vi "Day 4 - Scratchcards.vi"() -> ()   [LabVIEW 2020, in "AoC 2023.lvlib"]
uses:
  AoC 2023.lvlib
  <vilib>/Utility/miscctls.llb/LVMapReplaceAction.ctl
  0a7cd956-c678-4c40-ba95-56d0818c301c.vi
  3b086681-bc74-48f0-999b-988c14eea146.vi
  9d519f65-ef92-499d-aef6-91ab72298a4b.vi
  0a7cd956-c678-4c40-ba95-56d0818c301c.vi/7c7783df-fd5a-49d9-9b7a-63cc9fb0e4e5.vi
  3b086681-bc74-48f0-999b-988c14eea146.vi/7c7783df-fd5a-49d9-9b7a-63cc9fb0e4e5.vi
panel:
  out "Puzzle Part-2 Answer":string
  out "Puzzle Answer":string
  in  "Puzzle Input":string="Card 1: 41 48 83 86 17 | 83 86  6 31 17  9 48 53\nCard 2: 13 32 20 16 61 | 61 30 68 82 17 32 24 19\nCard 3:  1 21 53 59 44 | 69 82 63 72 16 21 14  1\nCard 4: 41 92 73 84 69 | 59 84 76 51 58  5 54 83\nCard 5: 87 83 26 28 32 | 88 30 70 12 93 22 82 36\nCard 6: 31 18 13 56 72 | 74 77 10 23 35 67 36 11"
  # "Enter the Puzzle Input and run the VI"
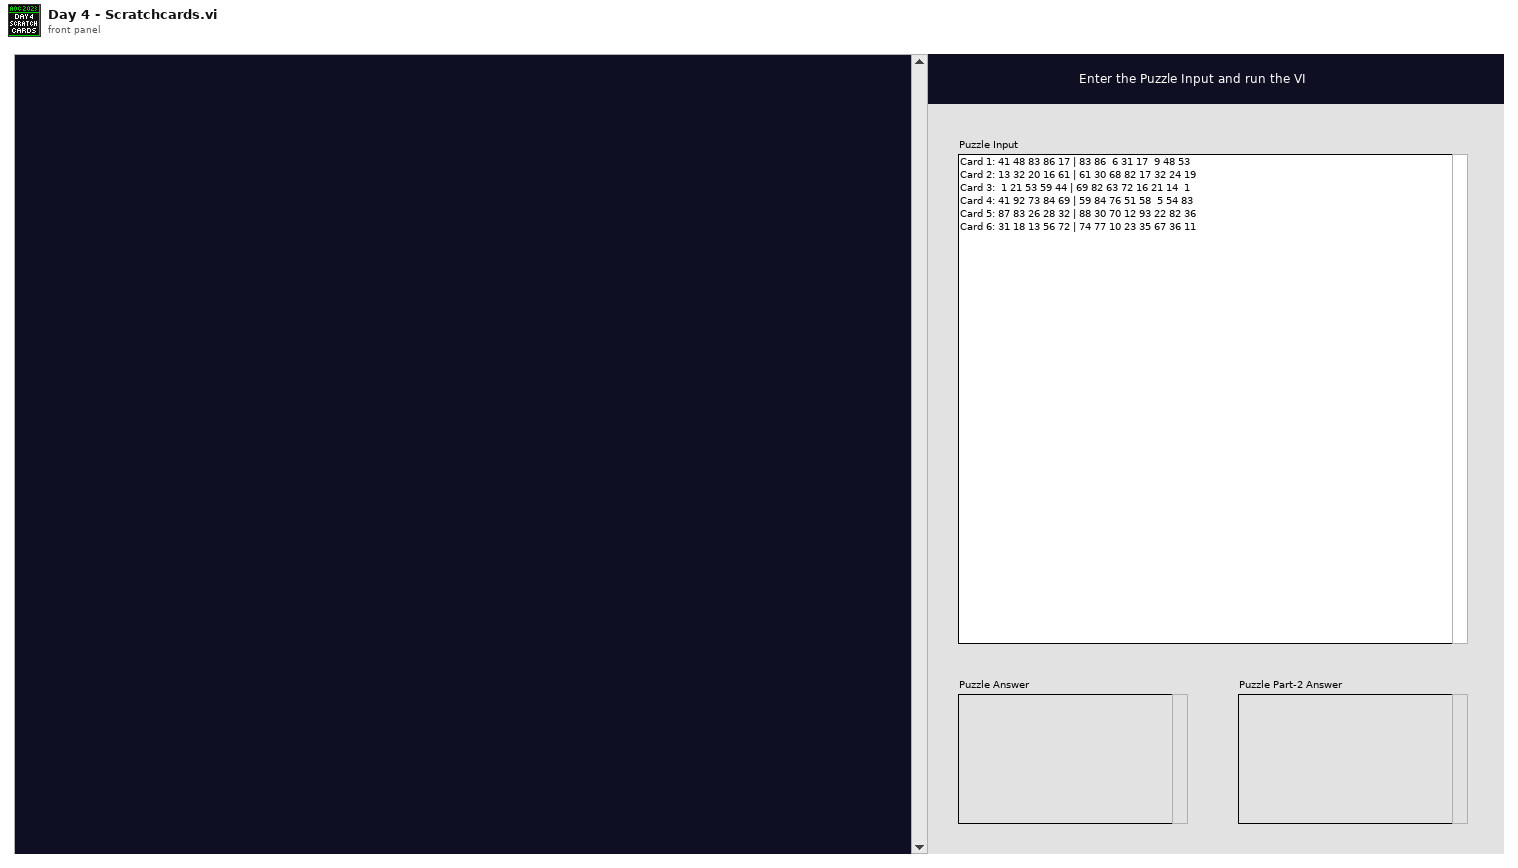
[diagram p1: front panel]
types:
  T1 = typedef "LVMapReplaceAction.ctl" = enum32{"Modify Entry only if found", "Add or Modify Entry", "Delete Entry"}
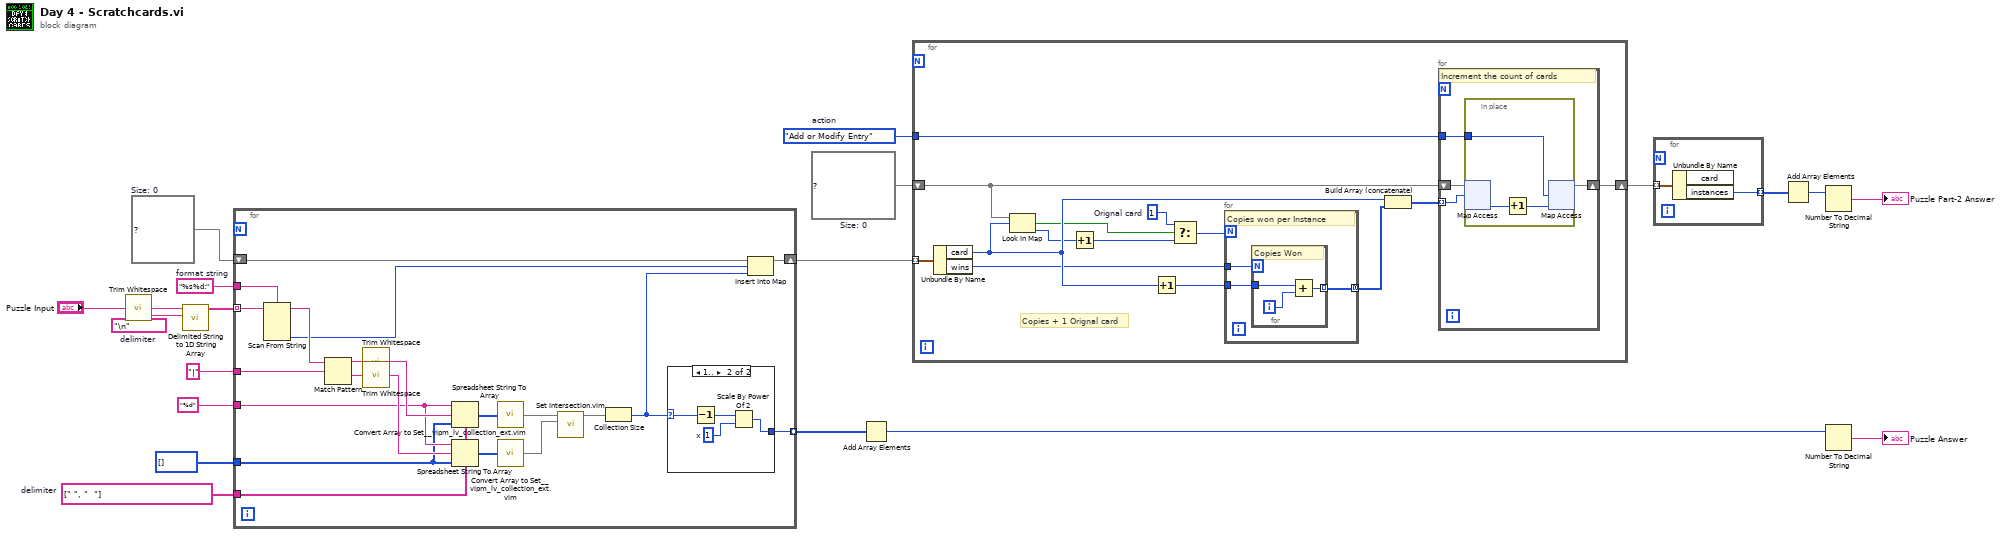
[diagram p0: block diagram]
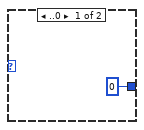
[diagram p2: hidden frame]
diagram:
  w1 = string[] [" ", "  "]  # delimiter
  w5 = map{i32, i32} {}  # Size: 0
  w6 = LVMapReplaceAction."Add or Modify Entry"  # action
  w8 = map{i32, i32} {}  # Size: 0
  w9 = "%s%d:"  # format string
  w17 = "\n"  # delimiter
  n1 = call <vilib>:"Trim Whitespace.vi"("string"="Puzzle Input") -> ("trimmed string"=w16:string)  [unwired: 1 in]
  n2 = call <vilib>:"Delimited String to 1D String Array.vi"("delimiter"=w17, "delimited string"=w16) -> ("string array"=w15:string[])  [unwired: 9 in]
  n3 = for {
    tunnel: w15 -> [w27] mode=indexing
    tunnel: "|" -> [w41]
    tunnel: "%d" -> [w31]
    shift-right: [w38] -> w7
    shift-left: w8 -> [w37]
    tunnel: [w34] -> w12 mode=indexing
    tunnel: i32[] [] -> [w30]
    tunnel: w9 -> [w26]
    tunnel: w1 -> [w21]
    n4 = Scan From String(format string=w26, input string=w27) -> (remaining string=w25:string, output 2=w22:i32)  [unwired: 5 in, 2 out]
    n5 = Match Pattern(string=w25, regular expression=w41) -> (before substring=w40:string, after substring=w39:string)  [unwired: 1 in, 2 out]
    n6 = call <vilib>:"Trim Whitespace.vi"("string"=w40) -> ("trimmed string"=w33:string)  [unwired: 1 in]
    n7 = call <vilib>:"Trim Whitespace.vi"("string"=w39) -> ("trimmed string"=w32:string)  [unwired: 1 in]
    n8 = Spreadsheet String To Array(delimiter (Tab)=w21, format string=w31, spreadsheet string=w33, array type (2D Dbl)=w30) -> (array=w29:i32[])
    n9 = Spreadsheet String To Array(delimiter (Tab)=w21, format string=w31, spreadsheet string=w32, array type (2D Dbl)=w30) -> (array=w28:i32[])
    n10 = call "Convert Array to Set__vipm_lv_collection_ext.vim"("array"=w29) -> ("set"=w36:set{i32})  [unwired: 6 in]
    n11 = call "Convert Array to Set__vipm_lv_collection_ext.vim"("array"=w28) -> ("set"=w35:set{i32})  [unwired: 6 in]
    n12 = call "Set Intersection.vim"("set 2"=w35, "set 1"=w36) -> ("intersection"=w24:set{i32})  [unwired: 9 in]
    n13 = Collection Size(1:w24) -> (0:w23:i32)
    n14 = case shown="1.." w23 {
      selector: w23 -> [_ w44]
      tunnel: [0 w46] -> w34
      frame ..0 {
      }
      frame 1.. {
        w45 = 1  # x
        n15 = Decrement(x=w44) -> (x-1=w43:i32)
        n16 = Scale By Power Of 2(n=w43, x=w45) -> (x*2^n=w46:i32)
      }
    }
    n17 = Insert Into Map(map in=w37, key=w22, value=w23) -> (map out=w38:map{i32, i32})  [unwired: 2 out]
  }
  n18 = Add Array Elements(numeric array=w12) -> (sum=w11:i32)
  n19 = for {
    tunnel: w7 -> [w60] mode=indexing
    tunnel: w6 -> [w59]
    shift-right: [w58] -> w4
    shift-left: w5 -> [w54]
    w49 = 1  # Orignal card
    # "Copies + 1 Orignal card"
    n20 = Unbundle By Name(w60) -> ("card"=w53:i32, "wins"=w52:i32)
    n21 = Look In Map(map=w54, key=w53) -> (key not found?=w50:bool, value=w48:i32)  [unwired: 1 in]
    n22 = Increment(x=w48) -> (x+1=w47:i32)
    n23 = Increment(x=w53) -> (x+1=w57:i32)
    n24 = Select(t=w49, s=w50, f=w47) -> (s? t:f=w51:i32)
    n25 = for {
      N: w51 -> [_]
      tunnel: w57 -> [w63]
      tunnel: [w62] -> w56 mode=concatenating
      tunnel: w52 -> [w61]
      # "Copies won per Instance"
      n26 = for {
        N: w61 -> [_]
        tunnel: w63 -> [w66]
        tunnel: [w64] -> w62 mode=indexing
        i -> [w65]
        # "Copies Won"
        n27 = Add(x=w66, y=w65) -> (x+y=w64:i32)
      }
    }
    n28 = Build Array (concatenate)(w53, w56) -> (w55:i32[])
    n29 = for {
      tunnel: w59 -> [w70]
      shift-right: [w69] -> w58
      shift-left: w54 -> [w68]
      tunnel: w55 -> [w67] mode=indexing
      # "Increment the count of cards"
      n30 = in-place {
        in-place-border: w70 -> [w71]
        n31 = in-place-map #1(w68, w67) -> (w73:i32)  [unwired: 1 in, 1 out]
        n32 = Increment(x=w73) -> (x+1=w72:i32)
        n33 = in-place-map #1(w72, w71) -> (w69:map{i32, i32})  [unwired: 2 out]
      }
    }
  }
  n34 = for {
    tunnel: w4 -> [w75] mode=indexing
    tunnel: [w74] -> w3 mode=indexing
    n35 = Unbundle By Name(w75) -> ("instances"=w74:i32)  [unwired: 1 out]
  }
  n36 = Add Array Elements(numeric array=w3) -> (sum=w2:i32)
  n37 = Number To Decimal String(number=w2) -> (decimal integer string=→"Puzzle Part-2 Answer":string)  [unwired: 1 in]
  n38 = Number To Decimal String(number=w11) -> (decimal integer string=→"Puzzle Answer":string)  [unwired: 1 in]
